vi "CircleCalculations-Ver1.vi"() -> ()   [LabVIEW 2018]
panel:
  in  "?":bool
  in  "?":bool
  out "Circumference":dbl format="%#_3g"
  out "Radius from Slider":dbl format="%#_2g"
  out "Area":dbl format="%#_4g"
  in  "Radius":dbl(slide) scale=0.0..10.0 scale format="%_2g"
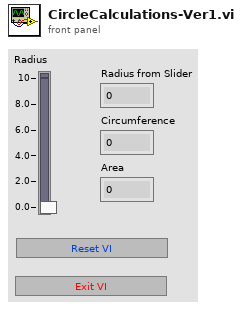
[diagram p1: front panel]
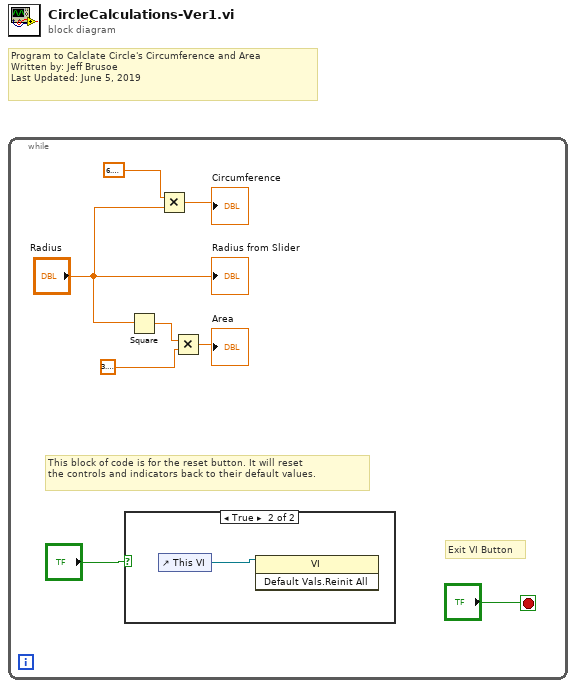
[diagram p0: block diagram]
diagram:
  # "Program to Calclate Circle's Circumference and Area\nWritten by: Jeff Brusoe\nLast Updated: June 5, 2019"
  n1 = while {
    stop <- "?" stop-if-true
    # "Exit VI Button"
    # "This block of code is for the reset button. It will reset\nthe controls and indicators back to their default values."
    n2 = case shown="True" "?" {
      frame False {
      }
      frame True {
        n3 = control-ref of="This VI"() -> (w9:refnum<vi>)
        n4 = invoke class="VI" method="Default Vals.Reinit All"(reference=w9) -> ()  [unwired: 2 in, 3 out]
      }
    }
    n5 = Square(x="Radius") -> (x^2=w6:dbl)
    n6 = Multiply(x=6.283185307179586, y="Radius") -> (x*y=→"Circumference":dbl)
    n7 = Multiply(x=w6, y=3.141592653589793) -> (x*y=→"Area":dbl)
    "Radius from Slider" <- "Radius"
  }
